vi "HIOKI PW3390 Hold.vi"(0 "VISA Resource":refnum<visa-resource-name>, 1 "Set/Query (F: Set)":bool, 5 "HOLD (0: OFF)":enum16{"OFF", "ON", "PEAK"}(ring), 11 "error in (no error)":errorcluster, 12 "OPC query (T: ON)":bool=TRUE, 13 "Error Out (F: Off)":bool) -> (4 "VISA Resource out":refnum<visa-resource-name>, 6 "HOLD out":enum16{"OFF", "ON", "PEAK"}(ring), 15 "error out":errorcluster={"status"=FALSE, "code"=1, "source"=""})   [LabVIEW 2009]
doc: "Set/Query\n Set: Send the setting commands for the device.\n Query: Query the setting of the device.\n\nHOLD\n Sets the HOLD status.\n\n<B>Note</B>\n Uses the \"HIOKI PW3390 TRG.vi\" to renew data during HOLD or PEAK HOLD status."
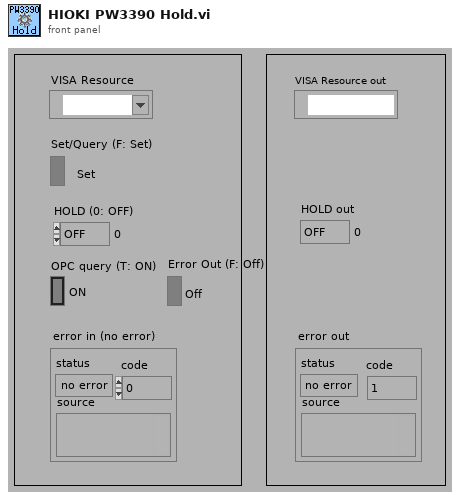
[diagram p1: front panel]
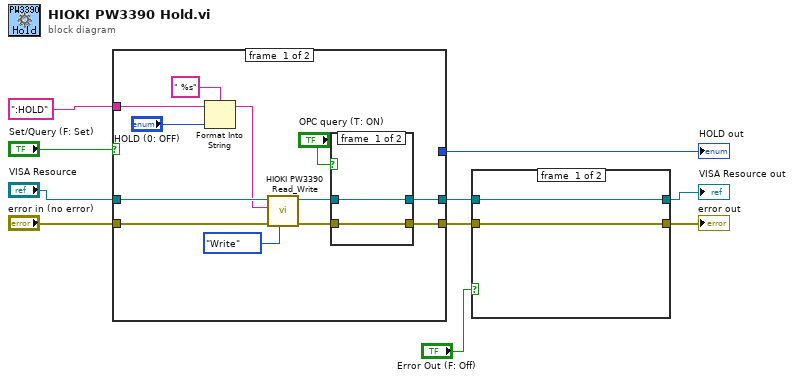
[diagram p0: block diagram]
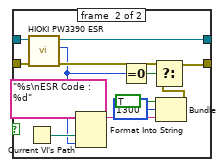
[diagram p2: hidden frame]
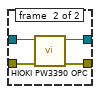
[diagram p3: hidden frame]
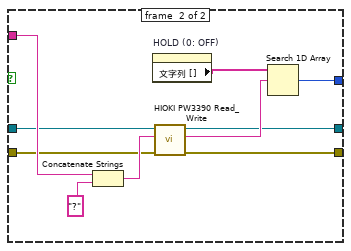
[diagram p4: hidden frame]
diagram:
  n1 = case shown="FALSE" "Set/Query (F: Set)" {
    tunnel: "error in (no error)" -> [w20 w30]
    tunnel: [w11 w32] -> w4
    tunnel: "VISA Resource" -> [w21 w29]
    tunnel: [w12 w33] -> w5
    tunnel: ":HOLD" -> [w18 w31]
    tunnel: [_ w37] -> w7
    frame #0 {
      n2 = Format Into String(format string=" %s", initial string=w18, "HOLD (0: OFF)") -> (resulting string=w17:string)  [unwired: 1 in, 1 out]
      n3 = call <instrlib>:"HIOKI PW3390 Read_Write.vi"("Read/Write"=enum16{"Read", "Write"}."Write", "error in (no error)"=w20, "data in"=w17, "VISA Resource"=w21) -> ("error out"=w13:errorcluster, "VISA Resource out"=w14:refnum<visa-resource-name>)  [unwired: 5 in, 1 out]
      n4 = case shown="TRUE" "OPC query (T: ON)" {
        tunnel: [w24 w28] -> w12
        tunnel: [w23 w27] -> w11
        tunnel: w14 -> [w24 w26]
        tunnel: w13 -> [w23 w25]
        frame #0 {
        }
        frame #1 {
          n5 = call <instrlib>:"HIOKI PW3390 OPC.vi"("error in (no error)"=w25, "VISA Resource"=w26) -> ("error out"=w27:errorcluster, "VISA Resource out"=w28:refnum<visa-resource-name>)  [unwired: 7 in, 1 out]
        }
      }
    }
    frame #1 {
      n6 = Concatenate Strings(w31, "?") -> (w36:string)
      n7 = property on="HOLD (0: OFF)" class="Enum (strict)"() -> ("文字列 []"=w35:string[])  [unwired: 2 in, 2 out]
      n8 = call <instrlib>:"HIOKI PW3390 Read_Write.vi"("error in (no error)"=w30, "data in"=w36, "VISA Resource"=w29) -> ("error out"=w32:errorcluster, "data out"=w34:string, "VISA Resource out"=w33:refnum<visa-resource-name>)  [unwired: 6 in]
      n9 = Search 1D Array(1D array=w35, element=w34) -> (index of element=w37:i32)  [unwired: 1 in]
    }
  }
  "HOLD out" <- w7
  n10 = case shown="TRUE" "Error Out (F: Off)" {
    tunnel: w5 -> [w40 w53]
    tunnel: w4 -> [w39 w52]
    tunnel: [w39 w42] -> w3
    tunnel: [w40 w51] -> w1
    frame #0 {
    }
    frame #1 {
      n11 = Current VI's Path() -> (path=w49:path)
      n12 = call <instrlib>:"HIOKI PW3390 ESR.vi"("error in (no error)"=w52, "VISA Resource"=w53) -> ("error out"=w43:errorcluster, "Output Value"=w41:u8, "VISA Resource out"=w51:refnum<visa-resource-name>)  [unwired: 6 in, 1 out]
      n13 = Format Into String(format string="%s\nESR Code : %d", w49, w41) -> (resulting string=w45:string)  [unwired: 2 in, 1 out]
      n14 = Equal To 0?(x=w41) -> (x = 0?=w50:bool)
      n15 = Bundle("status"=TRUE, "code"=1300, w45) -> (w44:cluster{"status":bool, "code":i32, string})  [unwired: 1 in]
      n16 = Select(t=w43, s=w50, f=w44) -> (s? t:f=w42:errorcluster)
    }
  }
  "error out" <- w3
  "VISA Resource out" <- w1
